vi "ClimbExecute_CtrlOnly.vi"(8 "Left Hard Limit Rev":bool, 9 "Left Sensor Position":dbl, 10 "Right Hard Limit Rev":bool, 11 "Right Sensor Position":dbl) -> (0 "Left Dmd":dbl, 1 "Left Output":dbl, 2 "Right Demand":dbl, 3 "Right Output":dbl, 4 "Left OnTarget":bool, 5 "Right OnTarget":bool)   [LabVIEW 2023]
uses:
  <vilib>/Rock Robotics/WPI/ThirdParty/JAS_Junk/TrajLib/VI/numCmd_ObtainQueue_OneDbl.vi
  <vilib>/Rock Robotics/WPI/ThirdParty/JAS_Junk/TrajLib/MathUtil_Clamp.vi
  <vilib>/Rock Robotics/WPI/ThirdParty/JAS_Junk/TrajLib/Trajectory_Library.lvlib
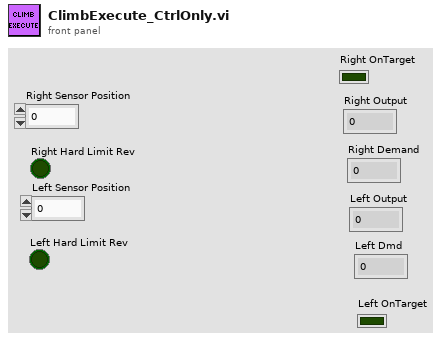
[diagram p1: front panel]
types:
  T1 = typedef "Trajectory_Library.lvlib/PosCtrl_Tuning_Type.ctl" = cluster{"Slope":dbl, "Offset":dbl, "Error Deadband":dbl, "At Reference Count":i32, "Negate Output":bool, "Max Allowd Position":dbl, "Min Allowd Position":dbl}
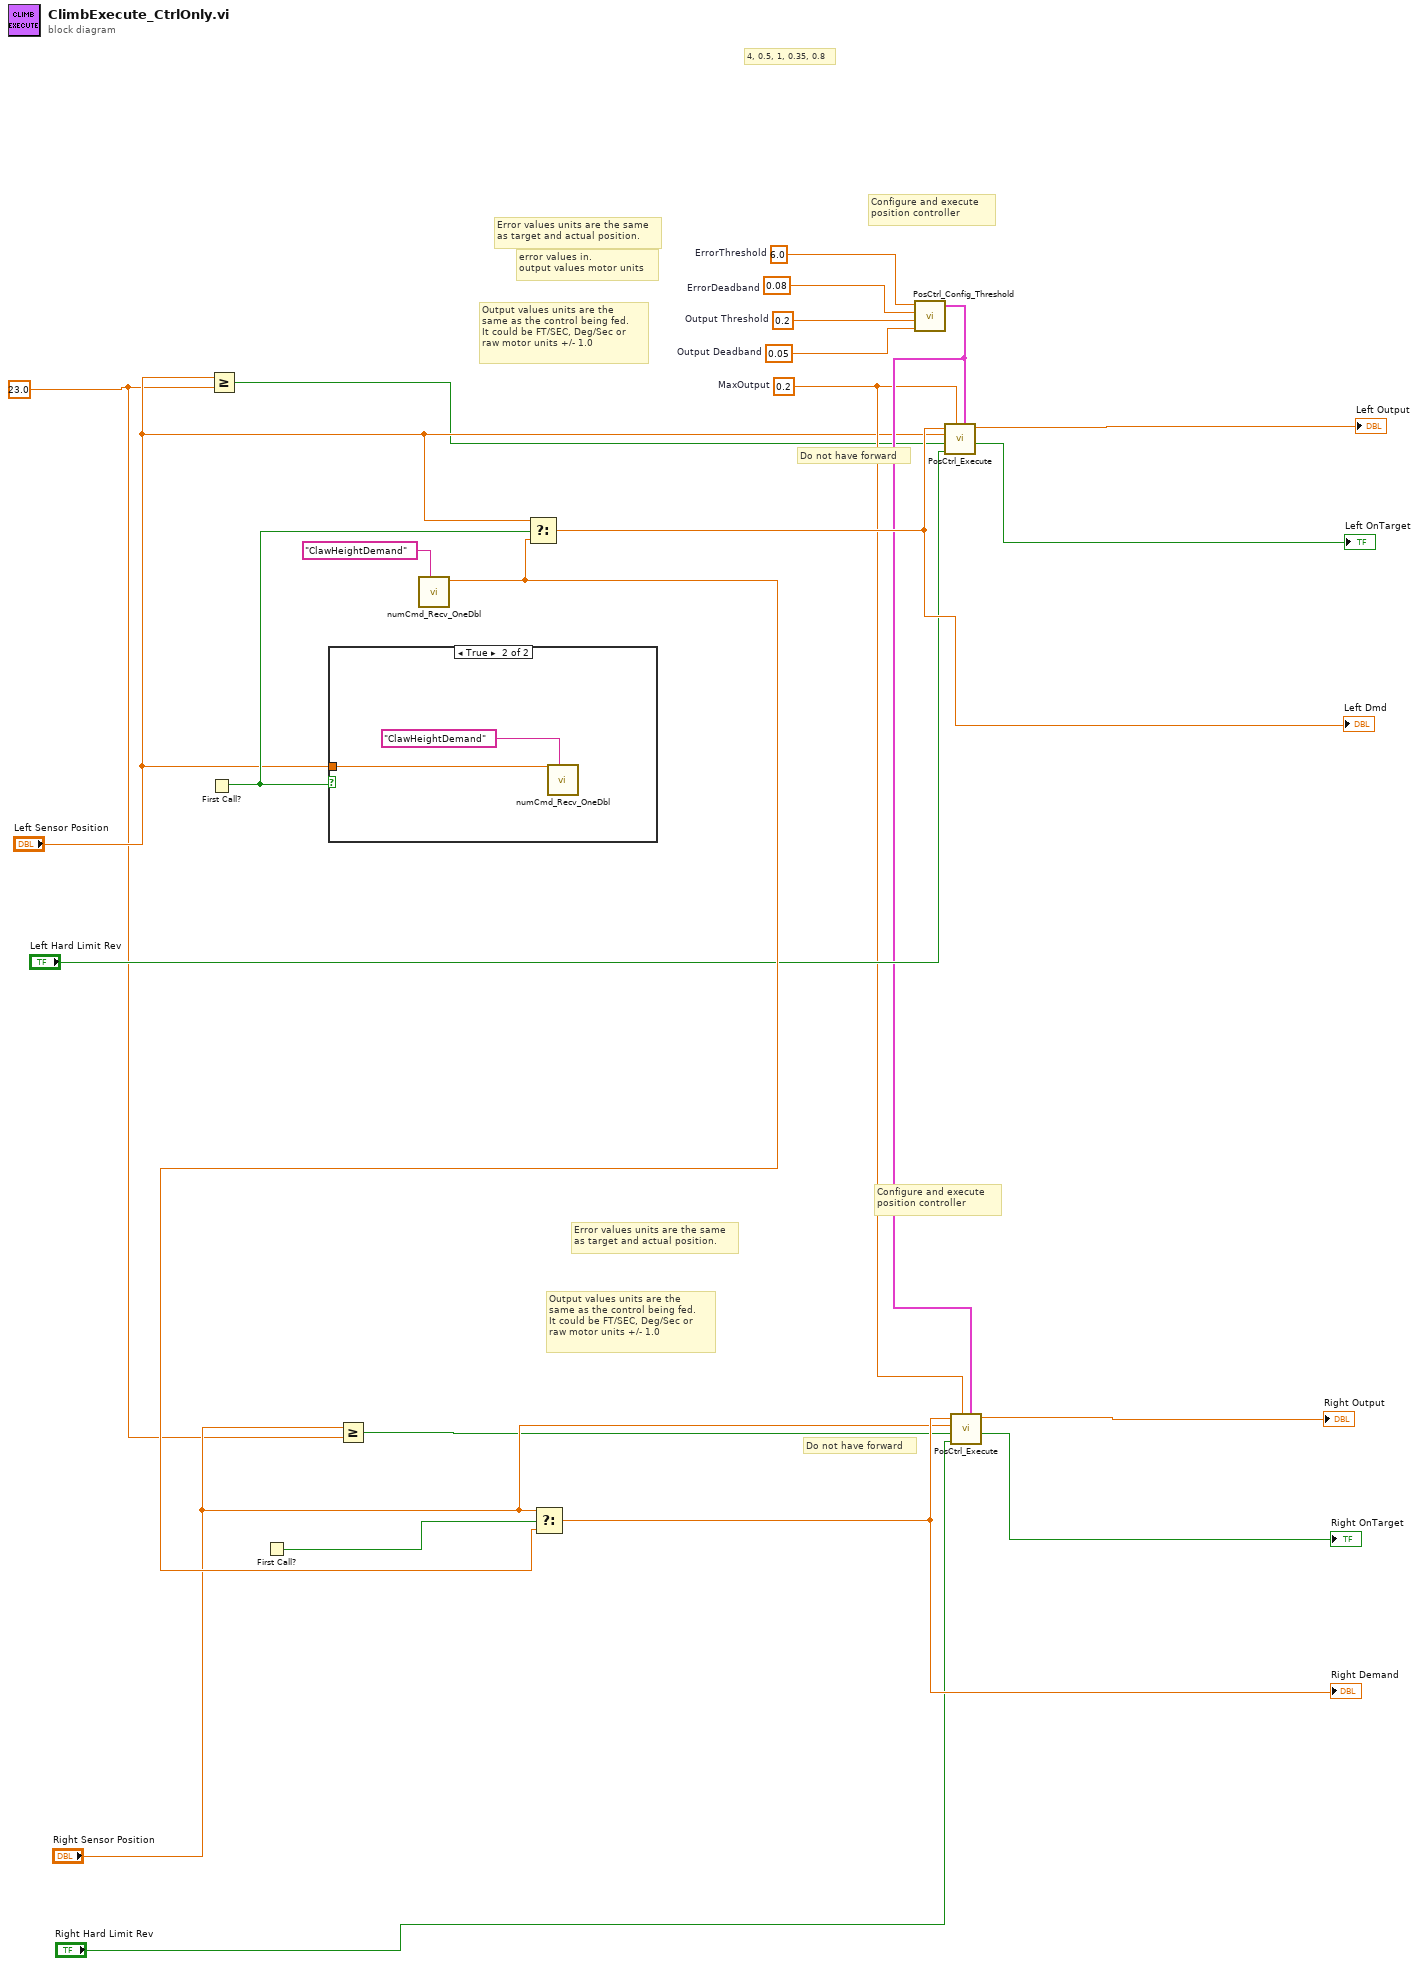
[diagram p0: block diagram]
diagram:
  w2 = 23.0 ("y")
  w6 = 0.2  # MaxOutput
  w23 = 6.0  # ErrorThreshold
  w22 = 0.08  # ErrorDeadband
  w21 = 0.2  # Output Threshold
  w20 = 0.05  # Output Deadband
  # "4, 0.5, 1, 0.35, 0.8"
  # "error values in.\noutput values motor units"
  # "Do not have forward"
  # "Output values units are the\nsame as the control being fed.  \nIt could be FT/SEC, Deg/Sec or\nraw motor units +/- 1.0"
  # "Error values units are the same \nas target and actual position."
  # "Configure and execute \nposition controller"
  # "Do not have forward"
  # "Output values units are the\nsame as the control being fed.  \nIt could be FT/SEC, Deg/Sec or\nraw motor units +/- 1.0"
  # "Error values units are the same \nas target and actual position."
  # "Configure and execute \nposition controller"
  n1 = First Call?() -> (First Call?: T/F=w19:bool)
  n2 = Greater Or Equal?(x="Left Sensor Position", y=w2) -> (x >= y?=w4:bool)
  n3 = First Call?() -> (First Call?: T/F=w14:bool)
  n4 = case shown="True" w19 {
    tunnel: "Left Sensor Position" -> [_ w24]
    frame False {
    }
    frame True {
      n5 = call <vilib>:"numCmd_Recv_OneDbl.vi"("Command Name"="ClawHeightDemand", "Initial Value"=w24) -> ()  [unwired: 7 in, 3 out]
    }
  }
  n6 = Greater Or Equal?(x="Right Sensor Position", y=w2) -> (x >= y?=w1:bool)
  n7 = call <vilib>:"numCmd_Recv_OneDbl.vi"("Command Name"="ClawHeightDemand") -> ("Value"=w10:dbl)  [unwired: 8 in, 2 out]
  n8 = Select(t="Left Sensor Position", s=w19, f=w10) -> (s? t:f=w17:dbl)
  "Left Dmd" <- w17
  n9 = Select(t="Right Sensor Position", s=w14, f=w10) -> (s? t:f=w13:dbl)
  "Right Demand" <- w13
  n10 = call <vilib>:"PosCtrl_Config_Threshold.vi"("Output Deadband"=w20, "Output Threshold"=w21, "ErrorDeadband"=w22, "ErrorThreshold"=w23) -> ("PosCtrl_Config_Params"=w7:T1)  [unwired: 7 in]
  n11 = call <vilib>:"PosCtrl_Execute.vi"("PosCtrl_Config_Params"=w7, "MaxOutput"=w6, "Rev Limit Switch"="Left Hard Limit Rev", "Fwd Limit Switch"=w4, "CurrentPosition"="Left Sensor Position", "TargetPosition"=w17) -> ("OnTarget"=→"Left OnTarget":bool, "Output"=→"Left Output":dbl)  [unwired: 3 in, 1 out]
  n12 = call <vilib>:"PosCtrl_Execute.vi"("PosCtrl_Config_Params"=w7, "MaxOutput"=w6, "Rev Limit Switch"="Right Hard Limit Rev", "Fwd Limit Switch"=w1, "CurrentPosition"="Right Sensor Position", "TargetPosition"=w13) -> ("OnTarget"=→"Right OnTarget":bool, "Output"=→"Right Output":dbl)  [unwired: 3 in, 1 out]
